vi "InitModule1212(Host).vi"(0 "FPGA 1212 VI Reference":refnum<k20>, 1 "RIO Device IN":T1="RIO0" caption="RIO Device", 2 "CLOCK SELECTION":u8(ring) items=["Internal", "External (From SMA)"], 3 "INTERNAL CLOCK":u8(ring) items=["From Oscillator", "From FPGA Clock"], 4 "Master":bool=TRUE, 5 "error in":errorcluster, 6 "DCI IN":u32=38 max=332, 7 "Freq (Hz)":dbl=1250000000.0 format="%#_6p") -> (10 "DAC A Aligned":bool, 11 "FPGA DCM LOCKED":bool, 12 "DAC B Aligned":bool, 14 "FPGA VI Reference Out":refnum<k20>, 15 "RIO Device out":T1, 16 "DCI OUT":u32=38 max=332, 19 "error out":errorcluster)   [LabVIEW 2018]
uses:
  <vilib>/userdefined/High Color/nirio_resource_hc.ctl
  <vilib>/FPGAPlugInAG/Dynamic/niLvFpga_Close_Dynamic.vi
  <vilib>/rvi/interface/nirviCloseFPGA/nirviCloseFPGA.xnode
panel:
  out "Ps_Tap OUT":dbl=10.0
  out "DCI Array":u32[][](array[numeric])
  out "Retry":i32[](array[numeric])
  out "MULocked":u8[](array[numeric])
  in  "DEBUG":bool
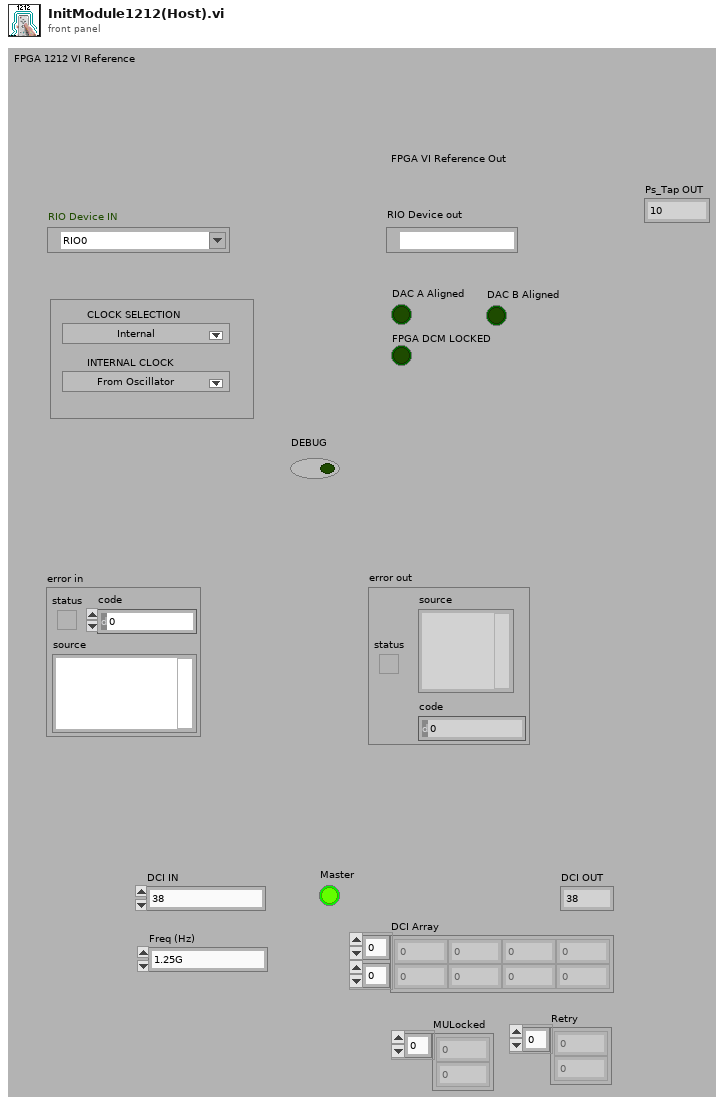
[diagram p1: front panel]
types:
  T1 = typedef "nirio_resource_hc.ctl" = tag
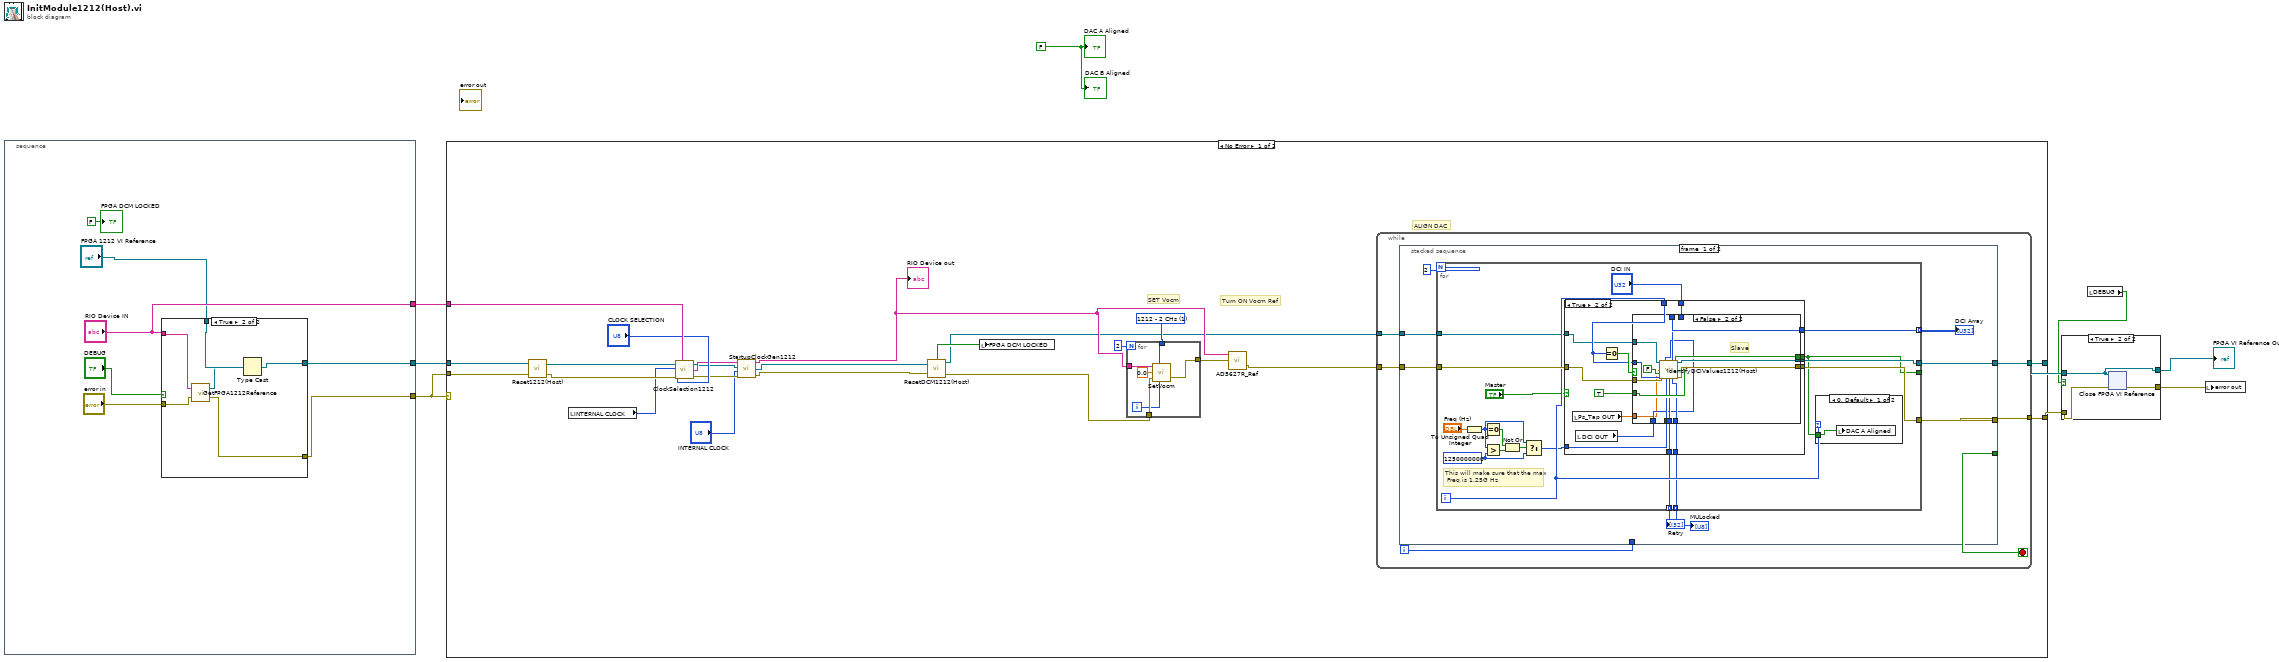
[diagram p0: block diagram]
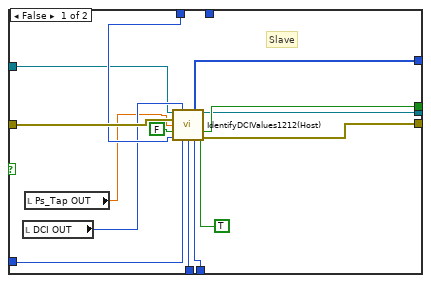
[diagram p3: hidden frame]
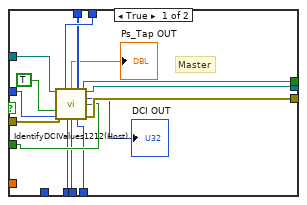
[diagram p4: hidden frame]
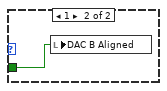
[diagram p5: hidden frame]
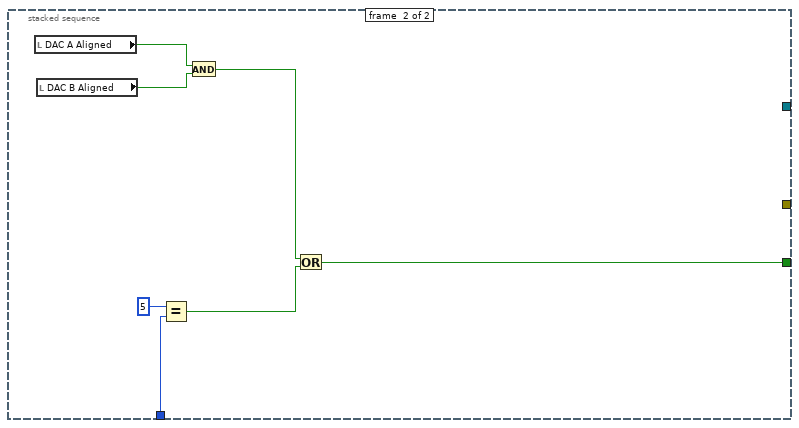
[diagram p6: hidden frame]
diagram:
  w9 = FALSE ("MULTI MODULE ALIGNED")
  n1 = stacked-sequence {
    tunnel: ["RIO Device IN"] -> w8
    tunnel: [w15] -> w7
    tunnel: [w11] -> w3
    frame #0 {
      n2 = case shown="True" "DEBUG" {
        tunnel: "RIO Device IN" -> [_ w22]
        tunnel: [w18 w19] -> w11
        tunnel: "error in" -> [w18 w21]
        tunnel: [w17 w23] -> w15
        tunnel: "FPGA 1212 VI Reference" -> [w17 w24]
        frame False {
        }
        frame True {
          n3 = call "GetFPGA1212Reference.vi"("error in"=w21, "RIO Device IN"=w22) -> ("error out"=w19:errorcluster, "FPGA VI Reference Out"=w20:refnum<k20>)
          n4 = Type Cast(type=w24, x=w20) -> (*(type *) &x=w23:refnum<k20>)
        }
      }
      "FPGA DCM LOCKED" <- FALSE ("FPGA DCM LOCKED")
    }
  }
  n5 = case shown="No Error" w3 {
    tunnel: w8 -> [w44 _]
    tunnel: w7 -> [w42 w154]
    tunnel: [w37 w154] -> w6
    tunnel: [w36 w153] -> w5
    tunnel: w3 -> [w35 w153]
    frame No Error {
      w39 = u8 1 items=["1120 - 1 CH", "1212 - 2 CHs"] ("ADAPTER NAME")
      # "ALIGN DAC"
      # "Turn ON Vocm Ref"
      # "SET Vocm"
      n6 = call "Reset1212(Host).vi"("error in"=w35, "FPGA Interface In"=w42) -> ("error out"=w46:errorcluster, "FPGA Interface Out"=w45:refnum<k20>)
      n7 = local read "INTERNAL CLOCK"() -> (w34:u8)
      n8 = call "ClockSelection1212.vi"("FPGA Interface In"=w45, "INTERNAL CLOCK"=w34, "CLOCK SELECTION"="CLOCK SELECTION", "error in (no error)"=w46, "RIO Device"=w44) -> ("FPGA Interface Out"=w31:refnum<k20>, "RIO Device out"=w32:T1, "error out"=w30:errorcluster)
      n9 = call "StartupClockGen1212.vi"("error in (no error)"=w30, "INTERNAL CLOCK"="INTERNAL CLOCK", "FPGA Interface In"=w31, "RIO Device"=w32) -> ("error out"=w26:errorcluster, "FPGA Interface Out"=w27:refnum<k20>, "RIO Device out"=w28:T1)
      "RIO Device out" <- w28
      n10 = call "ResetDCM1212(Host).vi"("error in"=w26, "FPGA Interface In"=w27) -> ("error out"=w43:errorcluster, "LOCKED"=w33:bool, "FPGA Interface Out"=w25:refnum<k20>)
      n11 = local write "FPGA DCM LOCKED"(w33) -> ()
      n12 = for {
        N: 2 -> [_]
        tunnel: w28 -> [w53]
        tunnel: w43 -> [w51]
        tunnel: w39 -> [w50]
        tunnel: [w48] -> w38
        i -> [w49]
        n13 = call "SetVocm.vi"("RIO Device"=w53, "ADAPTER NAME"=w50, "Vocm Offset(V)"=0.0, "error in (no error)"=w51, "Selected Output"=w49) -> ("error out"=w48:errorcluster)  [unwired: 1 out]
      }
      n14 = call "AD5627R_Ref.vi"("error in (no error)"=w38, "RIO Device"=w28) -> ("error out"=w47:errorcluster)  [unwired: 2 in, 1 out]
      n15 = while {
        tunnel: w47 -> [w59]
        tunnel: [w58] -> w37
        tunnel: [w57] -> w36
        tunnel: w25 -> [w54]
        i -> [w56]
        stop <- w55 stop-if-true
        n16 = stacked-sequence {
          tunnel: w59 -> [w67 _]
          tunnel: [w65 _] -> w58
          tunnel: [w64 _] -> w57
          tunnel: w56 -> [_ w152]
          tunnel: [_ w148] -> w55
          tunnel: w54 -> [w60 _]
          frame #0 {
            n17 = for {
              N: 2 -> [_]
              tunnel: w67 -> [w84]
              tunnel: [w85] -> w65
              tunnel: [w81] -> _
              tunnel: [w83] -> w64
              tunnel: [w78] -> w61 mode=indexing
              tunnel: [w77] -> w63 mode=indexing
              tunnel: [w76] -> w62 mode=indexing
              tunnel: w60 -> [w75]
              i -> [w82]
              w71 = u64 1250000000 ("f")
              # "This will make sure that the max\n Freq is 1.25G Hz"
              n18 = To Unsigned Quad Integer(1:"Freq (Hz)") -> (0:w72:u64)
              n19 = Equal To 0?(x=w72) -> (x = 0?=w69:bool)
              n20 = Greater?(x=w72, y=w71) -> (0:w70:bool)
              n21 = Not Or(1:w70, 2:w69) -> (0:w68:bool)
              n22 = Select(t=w72, s=w68, f=w71) -> (s? t:f=w74:u64)
              n23 = case shown="True" "Master" {
                tunnel: [w96 w114] -> w85
                tunnel: w84 -> [w95 w113]
                tunnel: [w94 w112] -> w83
                tunnel: w82 -> [w93 w106]
                tunnel: [w97 w111] -> w81
                tunnel: "DCI IN" -> [_ w109]
                tunnel: w74 -> [w98 w108]
                tunnel: [w92 w105] -> w78
                tunnel: [w91 w104] -> w77
                tunnel: [w90 w103] -> w76
                tunnel: w75 -> [w87 w101]
                frame False {
                  # "Slave"
                  n24 = local read "DCI OUT"() -> (w88:u32)
                  n25 = local read "Ps_Tap OUT"() -> (w86:dbl)
                  n26 = call "IdentifyDCIValues1212(Host).vi"("FPGA Interface In"=w87, "DCI from  Master"=w88, "error in (no error)"=w95, "Ps_Tap from Master"=w86, "Reset DAC"=TRUE, "Master"=FALSE, "Selected DAC"=w93, "Freq"=w98) -> ("DCI Array"=w92:u32[], "FPGA Interface Out"=w96:refnum<k20>, "DAC ALIGNED"=w97:bool, "MU_LOST_LOCKED"=w91:u8, "RetryCounter"=w90:i32, "error out"=w94:errorcluster)  [unwired: 2 out]
                }
                frame True {
                  n27 = local read "Ps_Tap OUT"() -> (w100:dbl)
                  n28 = local read "DCI OUT"() -> (w102:u32)
                  n29 = Equal To 0?(x=w106) -> (x = 0?=w107:bool)
                  n30 = case shown="False" w107 {
                    tunnel: [w129 w143] -> w114
                    tunnel: w113 -> [w128 w142]
                    tunnel: [w127 w141] -> w112
                    tunnel: [w126 w140] -> w111
                    tunnel: TRUE ("Reset DAC") -> [w125 w139]
                    tunnel: w109 -> [w124 _]
                    tunnel: w108 -> [w123 w137]
                    tunnel: w106 -> [w121 w138]
                    tunnel: w102 -> [_ w133]
                    tunnel: [w119 w134] -> w105
                    tunnel: [w118 w136] -> w104
                    tunnel: [w117 w135] -> w103
                    tunnel: w101 -> [w116 w131]
                    tunnel: w100 -> [_ w130]
                    frame True {
                      # "Master"
                      n31 = call "IdentifyDCIValues1212(Host).vi"("FPGA Interface In"=w116, "DCI from  Master"=w124, "error in (no error)"=w128, "Reset DAC"=w125, "Master"=TRUE, "Selected DAC"=w121, "Freq"=w123) -> ("Ps_Tap OUT"=→"Ps_Tap OUT":dbl, "DCI Array"=w119:u32[], "FPGA Interface Out"=w129:refnum<k20>, "DCI OUT"=→"DCI OUT":u32, "DAC ALIGNED"=w126:bool, "MU_LOST_LOCKED"=w118:u8, "RetryCounter"=w117:i32, "error out"=w127:errorcluster)  [unwired: 1 in]
                    }
                    frame False {
                      # "Slave"
                      n32 = call "IdentifyDCIValues1212(Host).vi"("FPGA Interface In"=w131, "DCI from  Master"=w133, "error in (no error)"=w142, "Ps_Tap from Master"=w130, "Reset DAC"=w139, "Master"=FALSE, "Selected DAC"=w138, "Freq"=w137) -> ("DCI Array"=w134:u32[], "FPGA Interface Out"=w143:refnum<k20>, "DAC ALIGNED"=w140:bool, "MU_LOST_LOCKED"=w136:u8, "RetryCounter"=w135:i32, "error out"=w141:errorcluster)  [unwired: 2 out]
                    }
                  }
                }
              }
              n33 = case shown="0, Default" w82 {
                tunnel: w81 -> [w144 w145]
                frame 0, Default {
                  n34 = local write "DAC A Aligned"(w144) -> ()
                }
                frame 1 {
                  n35 = local write "DAC B Aligned"(w145) -> ()
                }
              }
            }
            "MULocked" <- w63
            "Retry" <- w62
            "DCI Array" <- w61
          }
          frame #1 {
            n36 = local read "DAC A Aligned"() -> (w147:bool)
            n37 = local read "DAC B Aligned"() -> (w146:bool)
            n38 = Equal?(x=5, y=w152) -> (x = y?=w149:bool)
            n39 = And(x=w147, y=w146) -> (x .and. y?=w150:bool)
            n40 = Or(x=w150, y=w149) -> (x .or. y?=w148:bool)
          }
        }
      }
    }
    frame Error {
    }
  }
  n41 = local read "DEBUG"() -> (w2:bool)
  n42 = case shown="True" w2 {
    tunnel: w6 -> [w155 w157]
    tunnel: w5 -> [w156 w158]
    tunnel: [w156 w159] -> w1
    tunnel: [w155 w157] -> w4
    frame False {
    }
    frame True {
      n43 = xnode "Close FPGA VI Reference"("FPGA VI Reference In"=w157, "error in"=w158) -> ("error out"=w159:errorcluster)
    }
  }
  "FPGA VI Reference Out" <- w4
  n44 = local write "error out"(w1) -> ()
  "DAC A Aligned" <- w9
  "DAC B Aligned" <- w9
